vi "niWLAN - 80211abgnRxRW_NAPA.vi"(1 "#Packets Received":i32[](array[numeric]), 2 "PowerLevel":dbl[](array[numeric]), 9 "Test Time":dbl, 11 "error in (no error)":errorcluster, 12 "RxTestParameters":T1 {"OFDM Data Rate (Mbps)" items=["6", "9", "12", "18", "24", "36", "48", "54"]; "DSSS Data Rate (Mbps)" items=["1", "2", "5.5 CCK", "5.5 PBCC", "11 CCK", "11 PBCC", "22", "33"]; "80211n PLCP Frame Format" items=["Mixed Format", "Greenfield Format"]}) -> ()   [LabVIEW 2011]
uses:
  TV/RW/Includes/WLAN - TV - RW - INC - RxTestParameters.ctl
  <vilib>/Utility/file.llb/Write To Spreadsheet File (string).vi
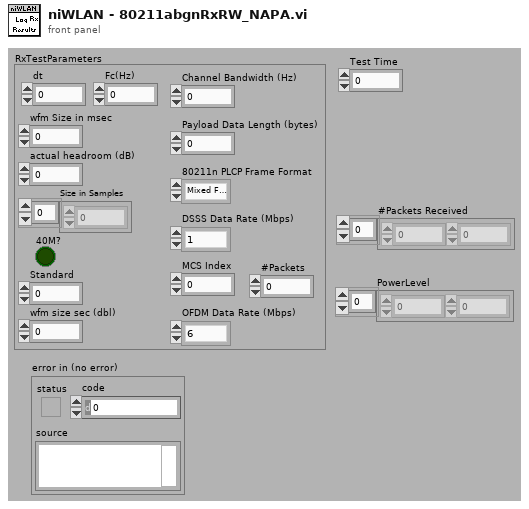
[diagram p1: front panel]
types:
  T1 = typedef "WLAN - TV - RW - INC - RxTestParameters.ctl" = cluster{"wfm Size in msec":i32, "actual headroom (dB)":dbl, "Size in Samples":i32[], "40M?":bool, "Standard ":i32, "wfm size sec (dbl)":dbl, "dt":dbl, "Channel Bandwidth (Hz)":dbl, "Payload Data Length (bytes)":i32, "80211n PLCP Frame Format":i32, "DSSS Data Rate (Mbps)":i32, "OFDM Data Rate (Mbps)":i32, "MCS Index":i32, "Fc(Hz)":dbl, "#Packets":i32}
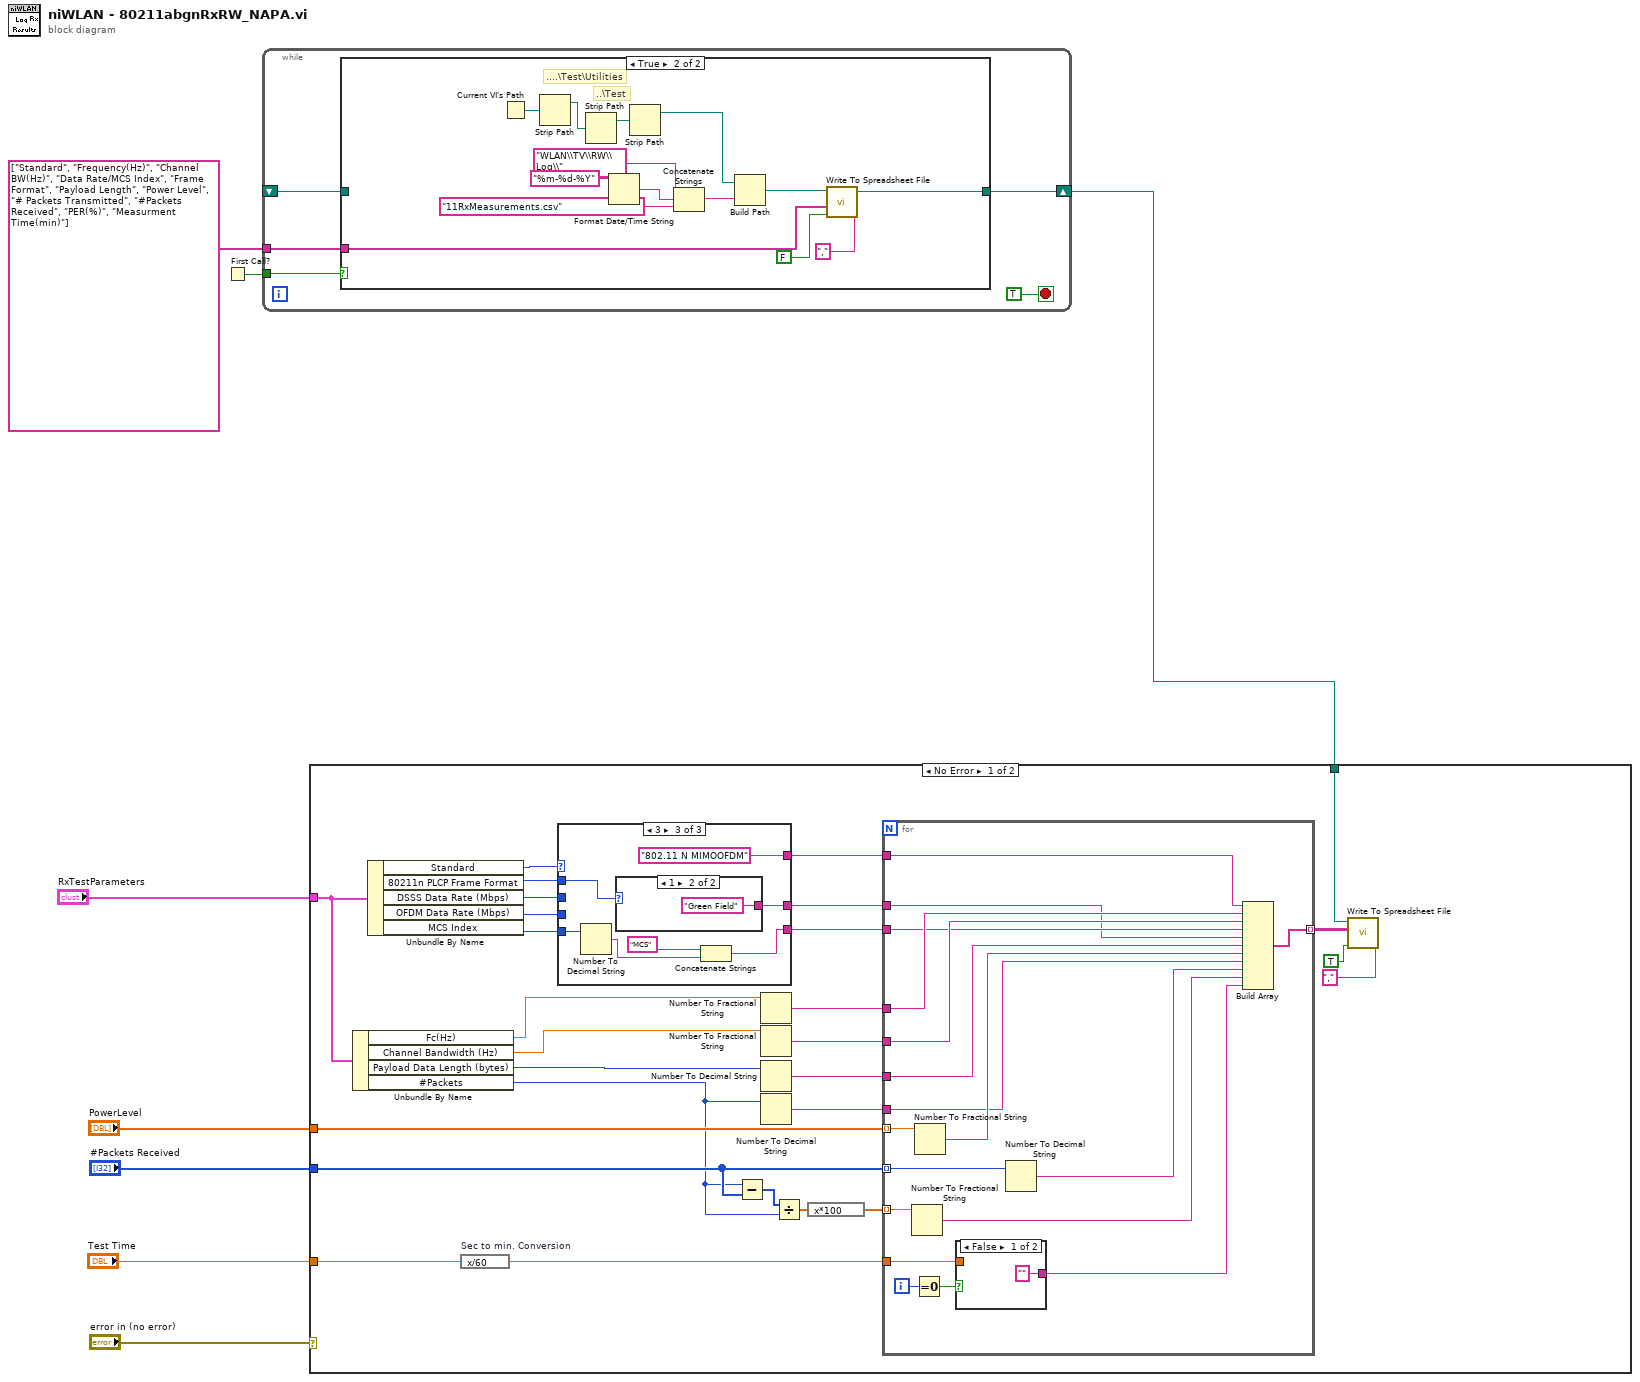
[diagram p0: block diagram]
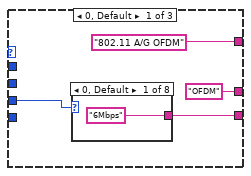
[diagram p3: hidden frame]
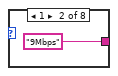
[diagram p4: hidden frame]
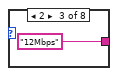
[diagram p5: hidden frame]
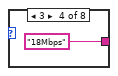
[diagram p6: hidden frame]
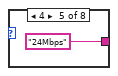
[diagram p7: hidden frame]
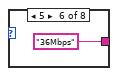
[diagram p8: hidden frame]
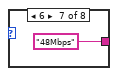
[diagram p9: hidden frame]
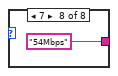
[diagram p10: hidden frame]
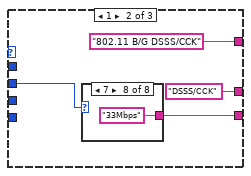
[diagram p11: hidden frame]
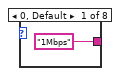
[diagram p12: hidden frame]
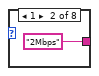
[diagram p13: hidden frame]
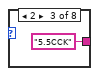
[diagram p14: hidden frame]
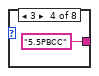
[diagram p15: hidden frame]
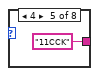
[diagram p16: hidden frame]
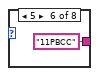
[diagram p17: hidden frame]
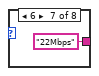
[diagram p18: hidden frame]
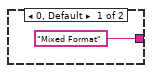
[diagram p19: hidden frame]
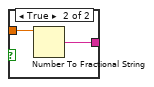
[diagram p20: hidden frame]
diagram:
  n1 = First Call?() -> (First Call?: T/F=w5:bool)
  n2 = while {
    tunnel: w5 -> [w12]
    shift-right: [w11] -> w4
    shift-left: _ -> [w10]
    tunnel: string[] ["Standard", "Frequency(Hz)", "Channel BW(Hz)", "Data Rate/MCS Index", "Frame Format", "Payload Length", "Power Level", "# Packets Transmitted", "#Packets Received", "PER(%)", "Measurment Time(min)"] -> [w9]
    stop <- TRUE stop-if-true
    n3 = case shown="True" w12 {
      tunnel: [w14 w16] -> w11
      tunnel: w10 -> [w14 _]
      tunnel: w9 -> [_ w15]
      frame False {
      }
      frame True {
        # "....\\Test\\Utilities"
        # "..\\Test"
        n4 = Current VI's Path() -> (path=w18:path)
        n5 = Strip Path(path=w18) -> (stripped path=w19:path)  [unwired: 1 out]
        n6 = Strip Path(path=w19) -> (stripped path=w20:path)  [unwired: 1 out]
        n7 = Format Date/Time String(time format string (%c)="%m-%d-%Y") -> (date/time string=w23:string)  [unwired: 2 in]
        n8 = Strip Path(path=w20) -> (stripped path=w24:path)  [unwired: 1 out]
        n9 = Concatenate Strings("WLAN\\TV\\RW\\Log\\" ("name or relative path"), w23, "11RxMeasurements.csv" ("name or relative path")) -> (w26:string)
        n10 = Build Path(base path=w24, name or relative path=w26) -> (appended path=w28:path)
        n11 = call-poly <vilib>:"Write To Spreadsheet File.vi"("delimiter (\\t)"="," ("delimiter (\\t)"), "append to file? (new file:F)"=FALSE, "1D data"=w15, "file path (dialog if empty)"=w28) -> ("new file path (Not A Path if cancelled)"=w16:path)  [unwired: 4 in]
      }
    }
  }
  n12 = case shown="No Error" "error in (no error)" {
    tunnel: w4 -> [w54 _]
    tunnel: "#Packets Received" -> [w33 _]
    tunnel: "RxTestParameters" -> [w48 _]
    tunnel: "Test Time" -> [w49 _]
    tunnel: "PowerLevel" -> [w36 _]
    frame No Error {
      n13 = Unbundle By Name(w48) -> ("Fc(Hz)"=w44:dbl, "Channel Bandwidth (Hz)"=w43:dbl, "Payload Data Length (bytes)"=w47:i32, "#Packets"=w32:i32)
      n14 = Unbundle By Name(w48) -> ("Standard"=w51:i32, "80211n PLCP Frame Format"=w50:i32, "DSSS Data Rate (Mbps)"=w39:i32, "OFDM Data Rate (Mbps)"=w40:i32, "MCS Index"=w38:i32)
      n15 = expression code="x/60" "Sec to min. Conversion"(w49) -> (w30:dbl)
      n16 = case shown="3" w51 {
        tunnel: ["802.11 A/G OFDM" "802.11 B/G DSSS/CCK" "802.11 N MIMOOFDM"] -> w52
        tunnel: w50 -> [_ _ w86]
        tunnel: ["OFDM" "DSSS/CCK" w85] -> w45
        tunnel: w40 -> [w58 _ _]
        tunnel: [w57 w70 w81] -> w37
        tunnel: w39 -> [_ w69 _]
        tunnel: w38 -> [_ _ w82]
        frame 0, Default {
          n17 = case shown="0, Default" w58 {
            tunnel: ["6Mbps" ("active channel") "9Mbps" ("active channel") "12Mbps" ("active channel") "18Mbps" ("active channel") "24Mbps" ("active channel") "36Mbps" ("active channel") "48Mbps" ("active channel") "54Mbps" ("active channel")] -> w57
            frame 0, Default {
            }
            frame 1 {
            }
            frame 2 {
            }
            frame 3 {
            }
            frame 4 {
            }
            frame 5 {
            }
            frame 6 {
            }
            frame 7 {
            }
          }
        }
        frame 1 {
          n18 = case shown="7" w69 {
            tunnel: ["1Mbps" ("active channel") "2Mbps" ("active channel") "5.5CCK" ("active channel") "5.5PBCC" ("active channel") "11CCK" ("active channel") "11PBCC" ("active channel") "22Mbps" ("active channel") "33Mbps" ("active channel")] -> w70
            frame 0, Default {
            }
            frame 1 {
            }
            frame 2 {
            }
            frame 3 {
            }
            frame 4 {
            }
            frame 5 {
            }
            frame 6 {
            }
            frame 7 {
            }
          }
        }
        frame 3 {
          n19 = Number To Decimal String(number=w82) -> (decimal integer string=w83:string)  [unwired: 1 in]
          n20 = case shown="1" w86 {
            tunnel: ["Mixed Format" "Green Field"] -> w85
            frame 0, Default {
            }
            frame 1 {
            }
          }
          n21 = Concatenate Strings("MCS" ("string"), w83) -> (w81:string)
        }
      }
      n22 = Subtract(x=w32, y=w33) -> (x-y=w34:i32[])
      n23 = Number To Fractional String(number=w44) -> (F-format string=w41:string)  [unwired: 3 in]
      n24 = Number To Fractional String(number=w43) -> (F-format string=w42:string)  [unwired: 3 in]
      n25 = Number To Decimal String(number=w47) -> (decimal integer string=w46:string)  [unwired: 1 in]
      n26 = Number To Decimal String(number=w32) -> (decimal integer string=w35:string)  [unwired: 1 in]
      n27 = Divide(x=w34, y=w32) -> (x/y=w31:dbl[])
      n28 = expression code="x*100"(w31) -> (w29:dbl[])
      n29 = for {
        tunnel: w52 -> [w101]
        tunnel: w30 -> [w102]
        tunnel: [w105] -> w53 mode=indexing
        tunnel: w46 -> [w100]
        tunnel: w45 -> [w96]
        tunnel: w42 -> [w98]
        tunnel: w41 -> [w99]
        tunnel: w37 -> [w97]
        tunnel: w33 -> [w95] mode=indexing
        tunnel: w36 -> [w94] mode=indexing
        tunnel: w35 -> [w93]
        tunnel: w29 -> [w91] mode=indexing
        i -> [w103]
        n30 = Number To Fractional String(number=w91) -> (F-format string=w90:string)  [unwired: 3 in]
        n31 = Equal To 0?(x=w103) -> (x = 0?=w104:bool)
        n32 = Number To Fractional String(number=w94) -> (F-format string=w107:string)  [unwired: 3 in]
        n33 = case shown="False" w104 {
          tunnel: ["" w110] -> w106
          tunnel: w102 -> [_ w109]
          frame False {
          }
          frame True {
            n34 = Number To Fractional String(number=w109) -> (F-format string=w110:string)  [unwired: 3 in]
          }
        }
        n35 = Number To Decimal String(number=w95) -> (decimal integer string=w92:string)  [unwired: 1 in]
        n36 = Build Array(w101, w99, w98, w97, w96, w100, w107, w93, w92, w90, w106) -> (w105:string[])
      }
      n37 = call-poly <vilib>:"Write To Spreadsheet File.vi"("delimiter (\\t)"="," ("delimiter (\\t)"), "append to file? (new file:F)"=TRUE, "2D data"=w53, "file path (dialog if empty)"=w54) -> ()  [unwired: 4 in, 1 out]
    }
    frame Error {
    }
  }
